vi "quaternion_rotate_vector.vi"(8 "Vector V":dbl[](array[numeric])=[0.2390633555184266, 0.3668401213238788, -0.04727309910073427] format="%#.5f", 11 "Q quaternion":dbl[](array[numeric])) -> (3 "Vector QVQ'":dbl[](array[numeric])=[0.2390633555184266, 0.3668401213238788, -0.04727309910073427] format="%#.5f")   [LabVIEW 2012]
panel:
  # "Directly rotate vector V using quaternion Q.  If many vectors are to be transformed using the same quaternion, then it is somewhat more efficient to convert to a transform (quanternion_to_transform) and use that.  But if the transform is not otherwise needed, then it may be less confusing to use this VI and stick to a single rotation representation."
  # "w"
  # "x1"
  # "x2"
  # "x3"
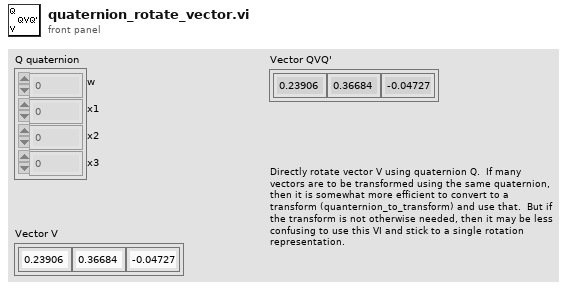
[diagram p1: front panel]
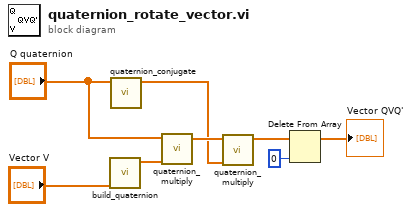
[diagram p0: block diagram]
diagram:
  n1 = call "build_quaternion.vi"("x"="Vector V") -> ("Quaternion"=w4:dbl[])  [unwired: 10 in]
  n2 = call "quaternion_conjugate.vi"("Q"="Q quaternion") -> ("Q conjugate"=w1:dbl[])  [unwired: 10 in]
  n3 = call "quaternion_multiply.vi"("q2"=w4, "q1"="Q quaternion") -> ("q1 * q2"=w5:dbl[])  [unwired: 9 in]
  n4 = call "quaternion_multiply.vi"("q2"=w1, "q1"=w5) -> ("q1 * q2"=w7:dbl[])  [unwired: 9 in]
  n5 = Delete From Array(array=w7, index=0) -> (array with subset deleted=→"Vector QVQ'":dbl[])  [unwired: 1 in, 1 out]
